vi "RDS Message Router.vi"(8 "error in (no error)":errorcluster, 10 "RDS Message":refnum<class "RDS Message.lvclass">, 11 "RDS Router Actor in":refnum<class "RDS Router Actor.lvclass">) -> (0 "error out":errorcluster, 3 "RDS Router Actor out":refnum<class "RDS Router Actor.lvclass">)   [LabVIEW 2015, in "RDS Abstracts.lvlib" / "RDS Router Actor.lvlib" / "RDS Router Actor.lvclass"]
uses:
  RDS Router Actor.lvclass
  Libraries/RDS Framework/RDS Message Class/RDS Message.lvclass
  RDS Router Actor.lvclass/RDS Router Actor.ctl
  RSD Subscription Class/RDS Router Subscription.lvclass
  RDS Parent Actor/RDS Parent Actor Messages/RDS Child Receive Message Msg/RDS Child Receive Message Msg.lvclass
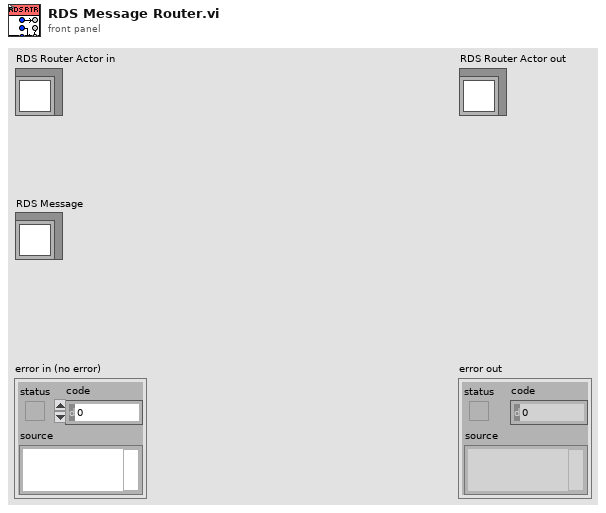
[diagram p1: front panel]
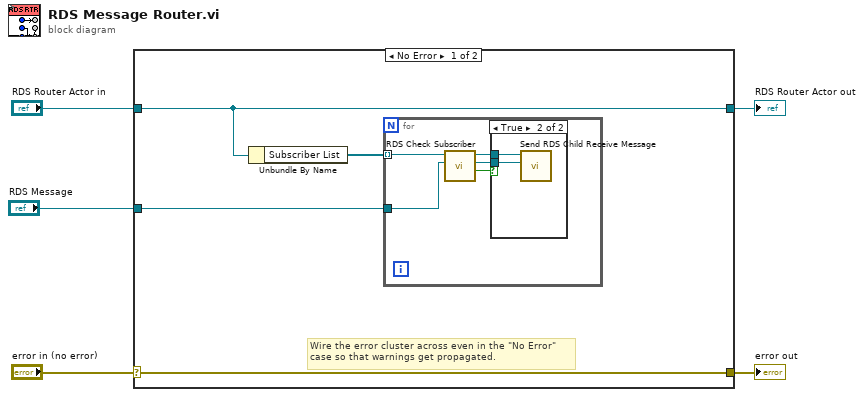
[diagram p0: block diagram]
diagram:
  n1 = case shown="No Error" "error in (no error)" {
    selector: "error in (no error)" -> [w9 w18]
    tunnel: [w9 w18] -> w4
    tunnel: [w8 w17] -> w2
    tunnel: "RDS Router Actor in" -> [w8 w17]
    tunnel: "RDS Message" -> [w6 _]
    frame No Error {
      # "Wire the error cluster across even in the \"No Error\"\ncase so that warnings get propagated."
      n2 = Unbundle By Name(w8) -> ("Subscriber List"=w7:refnum<class "RDS Router Subscription.lvclass">[])
      n3 = for {
        tunnel: w7 -> [w14] mode=indexing
        tunnel: w6 -> [w13]
        n4 = call "RDS Check Subscriber.vi"("RDS Message In"=w13, "RDS Router Subscription in"=w14) -> ("Subscribed?"=w12:bool, "RDS Message out"=w10:refnum<class "RDS Message.lvclass">, "RDS Child Enqueuer"=w11:refnum<class "Message Enqueuer.lvclass">)  [unwired: 6 in, 1 out]
        n5 = case shown="True" w12 {
          tunnel: w11 -> [_ w16]
          tunnel: w10 -> [_ w15]
          frame False {
          }
          frame True {
            n6 = call "Send RDS Child Receive Message.vi"("RDS Message"=w15, "Message Enqueuer in"=w16) -> ()  [unwired: 8 in, 2 out]
          }
        }
      }
    }
    frame Error {
    }
  }
  "error out" <- w4
  "RDS Router Actor out" <- w2
